vi "CALIBRATION_SUMMARY.vi"(0 "flow_slope_IN":dbl=50.0 format="%.2f", 1 "pressure_slope_IN":dbl=23.33 format="%.2f", 2 "DHT_Pressure_In":dbl=1.5 format="%.2f", 3 "Strip Path":bool, 4 "string_pot_slope_IN":dbl=1.5 format="%.2f", 5 "error in (no error)":errorcluster, 6 "flow_slope_OUT":dbl=56.0 format="%.2f", 7 "string_pot_slope_OUT":dbl=1.5 format="%.2f", 9 "Aux1_In":dbl=1.5 format="%.2f", 10 "Path":path=path "C:/KPRO_2010/Output_files/slopes-cal-record.txt", 11 "Aux2_In":dbl=1.5 format="%.2f", 12 "pressure_slope_OUT":dbl=23.33 format="%.2f", 13 "Aux3_In":dbl=1.5 format="%.2f", 17 "DHT_Pressure_In Offset":dbl=1.5 format="%.2f") -> (14 "Record Output Slopes for slopes.csv File":path, 15 "Record Output Slopes to  Record File":path, 19 "error out":errorcluster)   [LabVIEW 2016]
uses:
  <vilib>/Utility/file.llb/Read Delimited Spreadsheet (string).vi
  <vilib>/Utility/file.llb/Write Delimited Spreadsheet (string).vi
  Kpro Globals.vi
  <vilib>/Utility/file.llb/Write Delimited Spreadsheet (DBL).vi
panel:
  out "DHT_Pressure_Out Offset":dbl=1.5 format="%.2f"
  out "DHT_Pressure_Out":dbl=1.5 format="%.2f"
  out "Aux3_OUT":dbl=1.5 format="%.2f"
  out "Aux2_OUT":dbl=1.5 format="%.2f"
  out "Aux1_OUT":dbl=1.5 format="%.2f"
  out "first row":string[](array[string])
  out "Loop Counter":i32
  out "string_pot_slope_OUT 2":dbl=1.5 format="%.2f"
  out "string_pot_slope_IN 2":dbl=1.5 format="%.2f"
  out "KPRO Box Number":dbl=800.0
  out "Date_and_time":string
  out "pressure_slope_OUT 2":dbl=23.33 format="%.2f"
  out "flow_slope_OUT 2":dbl=51.35 format="%.2f"
  out "pressure_slope_IN 2":dbl=23.33 format="%.2f"
  out "flow_slope_IN 2":dbl=51.35 format="%.2f"
  in  "ok":bool
  # "CALIBRATION SUMMARY"
  # "Record these values in Kpro Box Calibration Log"
  # "DATE"
  # "TIME"
  # "Initial Slope              New Slope"
  # "Flow Sensor"
  # "mL/min/V"
  # "Up hole\nPressure Transducer"
  # "ft/V"
  # "ft/V"
  # "Down Hole Pressure\nTransducer Offset"
  # "Down Hole Pressure\nTransducer"
  # "Aux. Input 3"
  # "Aux. Input 2"
  # "Aux. Input 1"
  # "String Potentiometer"
  # "ft/V"
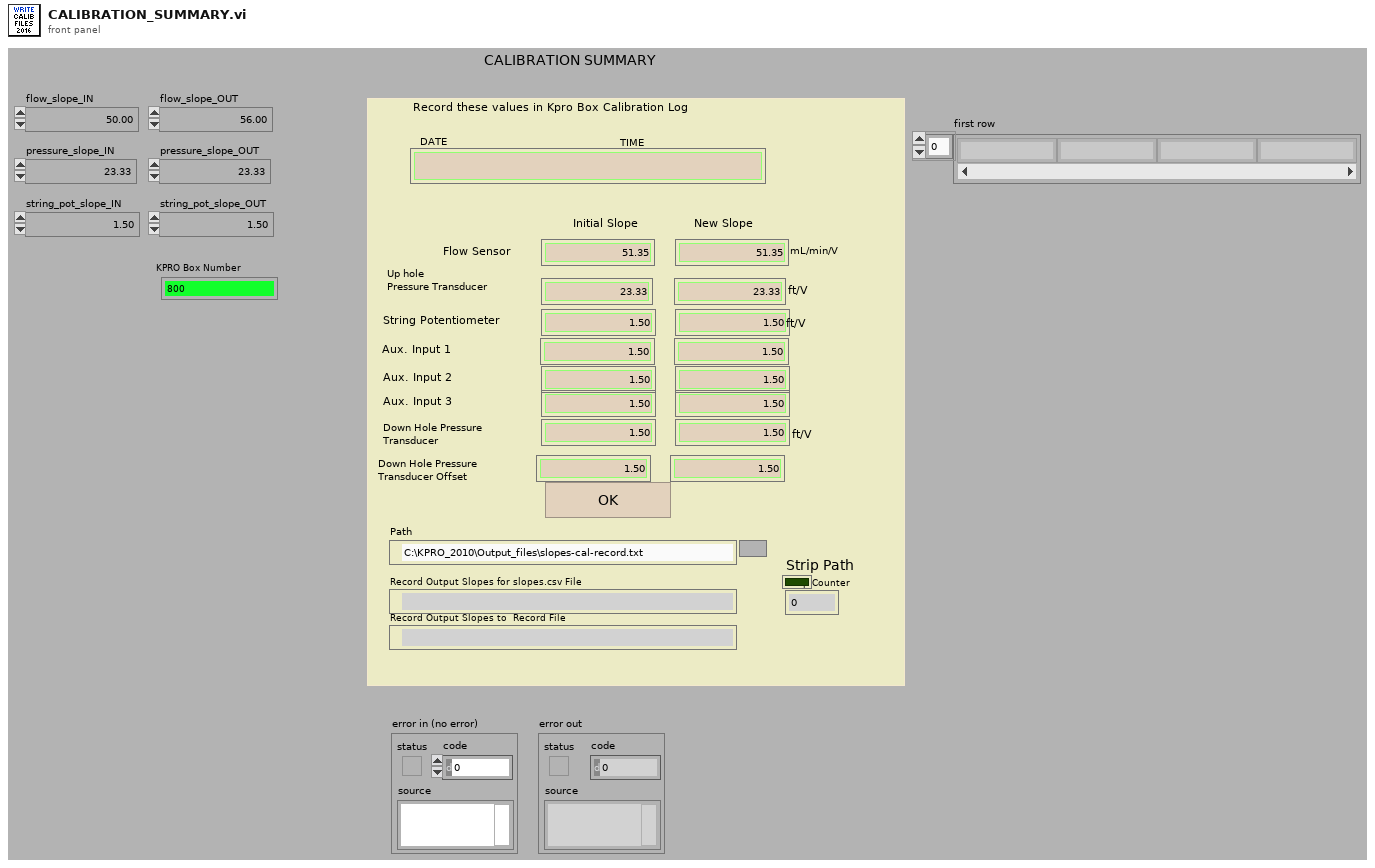
[diagram p1: front panel]
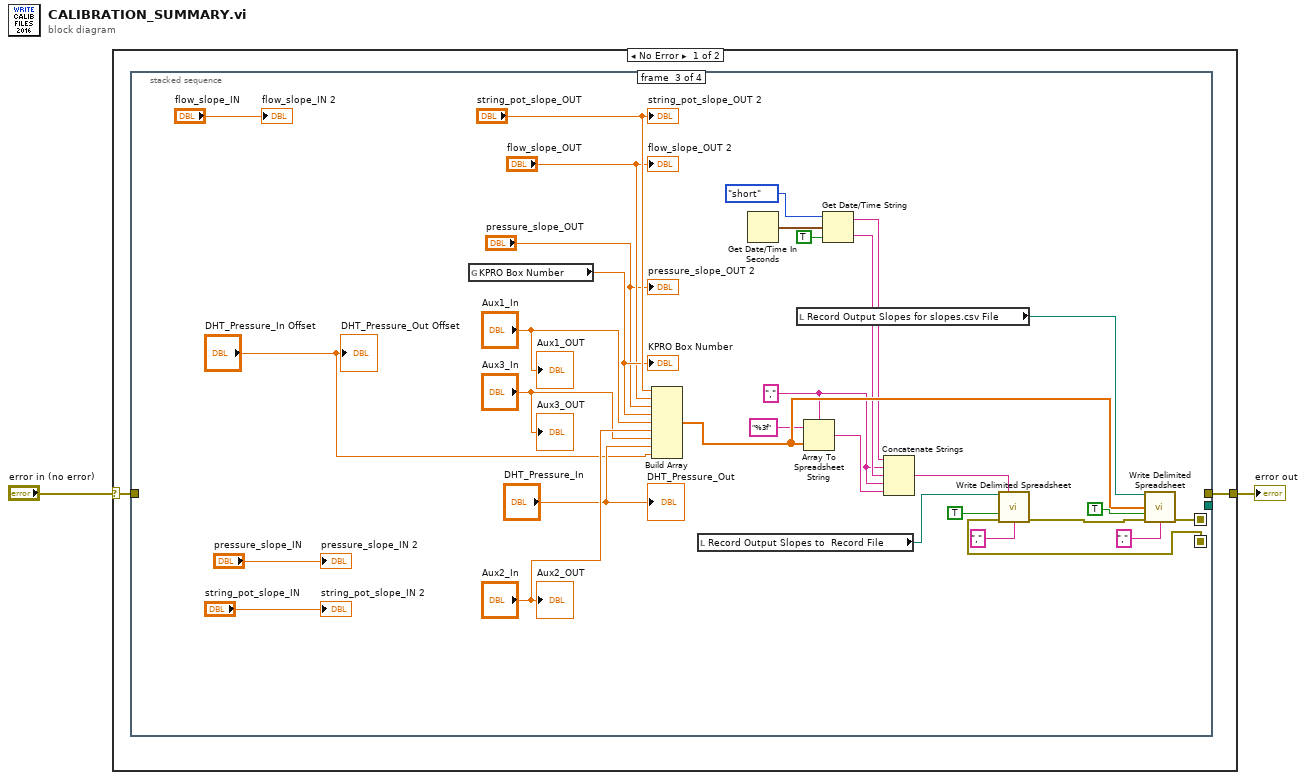
[diagram p0: block diagram]
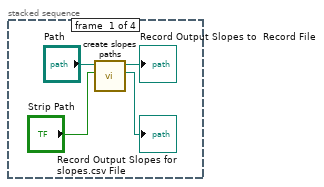
[diagram p2: hidden frame]
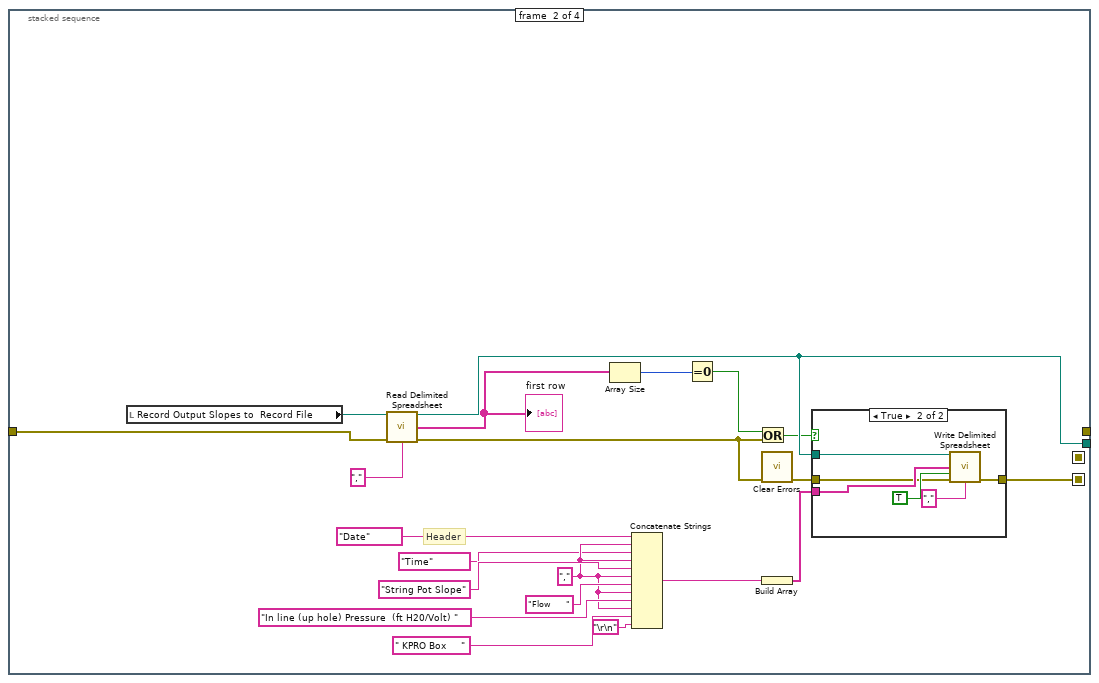
[diagram p3: hidden frame]
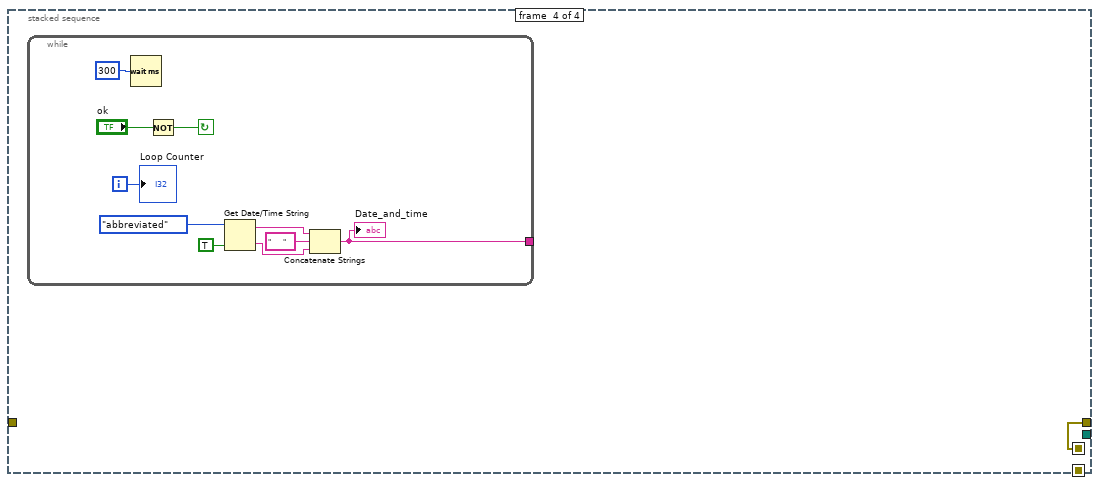
[diagram p5: hidden frame]
diagram:
  n1 = case shown="No Error" "error in (no error)" {
    selector: "error in (no error)" -> [w4 w79]
    tunnel: [w3 w79] -> w2
    frame No Error {
      n2 = stacked-sequence {
        seq-local: [_ w22 _ _] -> [_ _ w48 _]
        seq-local: [_ _ w59 _] -> [_ _ _ w68]
        tunnel: w4 -> [_ w16 _ _]
        tunnel: [_ _ _ w68] -> w3
        tunnel: [_ w17 _ _] -> _
        frame #0 {
          n3 = call "create slopes paths.vi"("Strip Path"="Strip Path", "Path"="Path") -> ("Record Output Slopes for slopes.csv File"=→"Record Output Slopes for slopes.csv File":path, "Record Output Slopes to  Record File"=→"Record Output Slopes to  Record File":path)  [unwired: 8 in]
        }
        frame #1 {
          w21 = "," ("string")
          # "Header"
          n4 = local read "Record Output Slopes to  Record File"() -> (w18:path)
          n5 = call-poly <vilib>:"Read Delimited Spreadsheet.vi"("file path (dialog if empty)"=w18, "error in (no error)"=w16, "delimiter (\\t)"="," ("delimiter (\\t)")) -> ("new file path (Not A Path if cancelled)"=w17:path, "first row"=w14:string[], "error out"=w10:errorcluster)  [unwired: 7 in, 3 out]
          "first row" <- w14
          n6 = Array Size(array=w14) -> (size(s)=w13:i32)
          n7 = Concatenate Strings("Date" ("string"), w21, "Time" ("string"), w21, "String Pot Slope" ("string"), w21, "Flow     " ("string"), w21, "In line (up hole) Pressure  (ft H20/Volt) " ("string"), w21, " KPRO Box     " ("string"), "\r\n") -> (w24:string)
          n8 = Equal To 0?(x=w13) -> (x = 0?=w11:bool)
          n9 = Or(x=w11, y=w10) -> (x .or. y?=w12:bool)
          n10 = call <vilib>:"Clear Errors.vi"("error in (no error)"=w10) -> ("error out"=w9:errorcluster)  [unwired: 5 in, 1 out]
          n11 = Build Array(w24) -> (w23:string[])
          n12 = case shown="True" w12 {
            tunnel: w23 -> [_ w35]
            tunnel: [w30 w34] -> w22
            tunnel: w17 -> [_ w32]
            tunnel: w9 -> [w30 w31]
            frame False {
            }
            frame True {
              n13 = call-poly <vilib>:"Write Delimited Spreadsheet.vi"("file path (dialog if empty)"=w32, "1D data"=w35, "append to file? (new file:F)"=TRUE, "error in (no error)"=w31, "delimiter (\\t)"="," ("delimiter (\\t)")) -> ("error out"=w34:errorcluster)  [unwired: 9 in, 1 out]
            }
          }
        }
        frame #2 {
          w43 = "," ("delimiter (\\t)")
          n14 = global read "Kpro Globals.vi" "KPRO Box Number"() -> (w62:dbl)
          "KPRO Box Number" <- w62
          n15 = Build Array("string_pot_slope_OUT", "flow_slope_OUT", "pressure_slope_OUT", w62, "Aux1_In", "Aux2_In", "Aux3_In", "DHT_Pressure_In", "DHT_Pressure_In Offset") -> (w53:dbl[])
          n16 = local read "Record Output Slopes to  Record File"() -> (w51:path)
          n17 = Get Date/Time In Seconds() -> (seconds since 1Jan1904=w55:timestamp)
          n18 = local read "Record Output Slopes for slopes.csv File"() -> (w58:path)
          n19 = Array To Spreadsheet String(delimiter (Tab)=w43, array=w53, 3:"%3f" ("format string")) -> (spreadsheet string=w44:string)
          n20 = Get Date/Time String(date format (0)=enum16{"short", "long", "abbreviated"}."short", seconds (now)=w55, want seconds? (F)=TRUE) -> (date string=w45:string, time string=w46:string)
          n21 = Concatenate Strings(w45, w43, w46, w43, w44) -> (w47:string)
          n22 = call-poly <vilib>:"Write Delimited Spreadsheet.vi"("file path (dialog if empty)"=w51, "format (%.3f)"=w47, "append to file? (new file:F)"=TRUE, "error in (no error)"=w48, "delimiter (\\t)"="," ("delimiter (\\t)")) -> ("error out"=w49:errorcluster)  [unwired: 9 in, 1 out]
          n23 = call-poly <vilib>:"Write Delimited Spreadsheet.vi"("file path (dialog if empty)"=w58, "1D data"=w53, "append to file? (new file:F)"=TRUE, "error in (no error)"=w49, "delimiter (\\t)"="," ("delimiter (\\t)")) -> ("error out"=w59:errorcluster)  [unwired: 9 in, 1 out]
          "pressure_slope_IN 2" <- "pressure_slope_IN"
          "flow_slope_IN 2" <- "flow_slope_IN"
          "string_pot_slope_IN 2" <- "string_pot_slope_IN"
          "pressure_slope_OUT 2" <- "pressure_slope_OUT"
          "flow_slope_OUT 2" <- "flow_slope_OUT"
          "string_pot_slope_OUT 2" <- "string_pot_slope_OUT"
          "Aux1_OUT" <- "Aux1_In"
          "Aux2_OUT" <- "Aux2_In"
          "Aux3_OUT" <- "Aux3_In"
          "DHT_Pressure_Out" <- "DHT_Pressure_In"
          "DHT_Pressure_Out Offset" <- "DHT_Pressure_In Offset"
        }
        frame #3 {
          n24 = while {
            tunnel: [w70] -> _
            i -> [w69]
            stop <- w78 continue-if-true
            n25 = Wait (ms)(milliseconds to wait=u32 300) -> ()  [unwired: 1 out]
            n26 = Not(x="ok") -> (.not. x?=w78:bool)
            n27 = Get Date/Time String(date format (0)=enum16{"short", "long", "abbreviated"}."abbreviated", want seconds? (F)=TRUE) -> (date string=w75:string, time string=w72:string)  [unwired: 1 in]
            n28 = Concatenate Strings(w75, "      " ("string"), w72) -> (w70:string)
            "Date_and_time" <- w70
            "Loop Counter" <- w69
          }
        }
      }
    }
    frame Error {
    }
  }
  "error out" <- w2
